vi "Download Dependencies.vi"(5 "Version":string, 7 "Target Directory":path, 8 "error in (no error)":errorcluster, 11 "Platform":T1) -> (0 "error out":errorcluster, 3 "Downloaded File":path)   [LabVIEW 2020, in "binary_installation_tools.lvlib"]
uses:
  binary_installation_tools.lvlib
  Binary Dependency Platform.ctl
  cc709fcc-8e9f-4311-8ae8-324c277baac9.vi
  Get Headers.vi
  <vilib>/security/Message Digest/API/Instances/File/SHA-256 File Checksum.vi
  <vilib>/httpClient/LabVIEWHTTPClient.lvlib
  <vilib>/security/Message Digest/API/NI_Message Digest API.lvlib
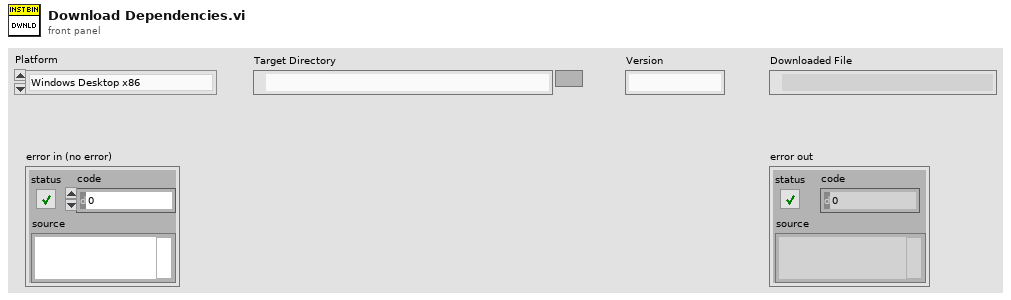
[diagram p1: front panel]
types:
  T1 = typedef "binary_installation_tools.lvlib/Binary Dependency Platform.ctl" = enum16{"Windows Desktop x86", "Windows Desktop x64", "Linux Desktop x64", "Linux Desktop aarch64", "NI Linux RT x64", "NI Linux RT armv7a"}
  T2 = enum16{"Get Manifest", "Check Download in Manifest", "Download", "Verify Checksum"}
  T3 = enum16{"Get Manifest", "Check Download in Manifest", "Download", "Verify Checksum"}[]
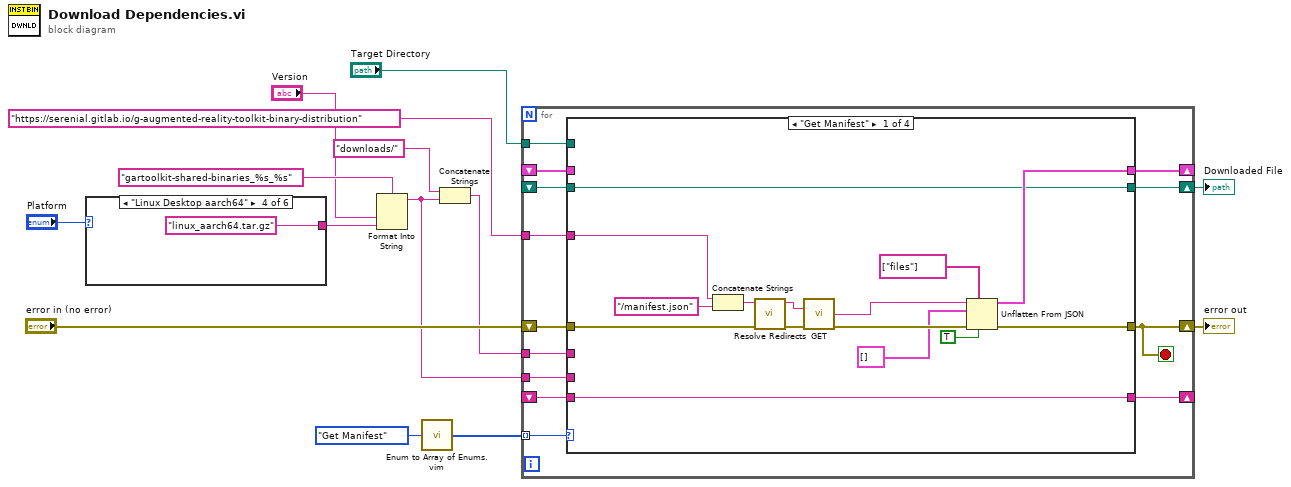
[diagram p0: block diagram]
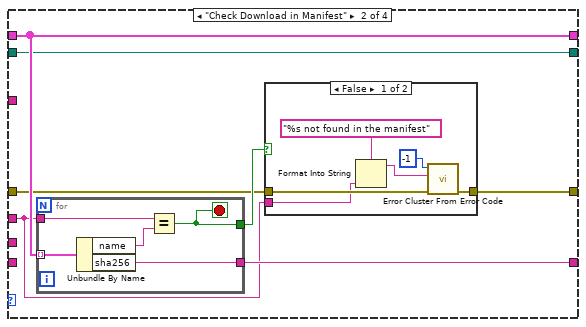
[diagram p2: hidden frame]
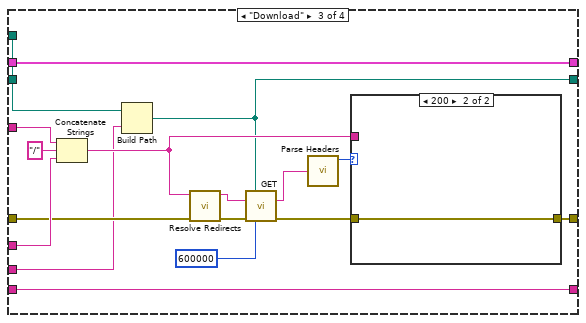
[diagram p4: hidden frame]
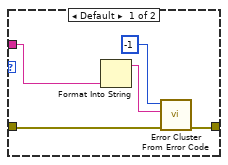
[diagram p5: hidden frame]
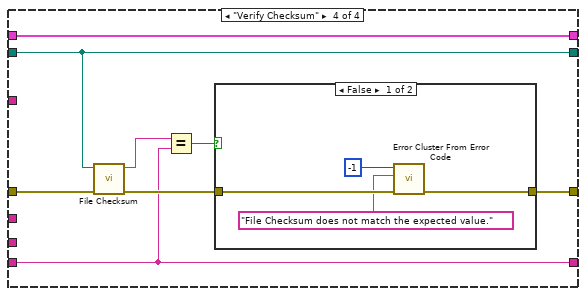
[diagram p6: hidden frame]
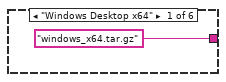
[diagram p8: hidden frame]
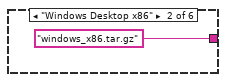
[diagram p9: hidden frame]
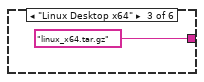
[diagram p10: hidden frame]
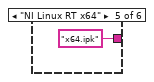
[diagram p11: hidden frame]
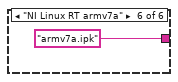
[diagram p12: hidden frame]
diagram:
  n1 = case shown="\"Linux Desktop aarch64\"" "Platform" {
    tunnel: ["windows_x64.tar.gz" "windows_x86.tar.gz" "linux_x64.tar.gz" "linux_aarch64.tar.gz" "x64.ipk" "armv7a.ipk"] -> w8
    frame "Windows Desktop x64" {
    }
    frame "Windows Desktop x86" {
    }
    frame "Linux Desktop x64" {
    }
    frame "Linux Desktop aarch64" {
    }
    frame "NI Linux RT x64" {
    }
    frame "NI Linux RT armv7a" {
    }
  }
  n2 = Format Into String(format string="gartoolkit-shared-binaries_%s_%s", "Version", w8) -> (resulting string=w4:string)  [unwired: 2 in, 1 out]
  n3 = call "Enum to Array of Enums.vim"("enum"=T2."Get Manifest") -> ("array of enums"=w11:T3)
  n4 = Concatenate Strings("downloads/" ("string"), w4) -> (w6:string)
  n5 = for {
    tunnel: w11 -> [w33] mode=indexing
    tunnel: "https://serenial.gitlab.io/g-augmented-reality-toolkit-binary-distribution" -> [w32]
    shift-right: [w25] -> w7
    shift-left: "error in (no error)" -> [w31]
    shift-right: [w30] -> _
    shift-left: _ -> [w29]
    tunnel: w6 -> [w28]
    shift-right: [w27] -> _
    shift-left: _ -> [w26]
    shift-right: [w24] -> w2
    shift-left: _ -> [w23]
    tunnel: w4 -> [w22]
    tunnel: "Target Directory" -> [w21]
    stop <- w25 stop-if-true
    n6 = case shown="\"Get Manifest\"" w33 {
      tunnel: w32 -> [w47 _ w81 _]
      tunnel: w31 -> [w44 w52 w78 w96]
      tunnel: [w38 w51 w72 w91] -> w25
      tunnel: [w36 w55 w84 w98] -> w30
      tunnel: w29 -> [_ w55 w84 w98]
      tunnel: w28 -> [_ w50 w80 _]
      tunnel: [w35 w54 w83 w93] -> w27
      tunnel: w26 -> [w35 _ w83 w93]
      tunnel: [w34 w49 w70 w97] -> w24
      tunnel: w23 -> [w34 w49 _ w97]
      tunnel: w22 -> [_ _ w69 _]
      tunnel: w21 -> [_ _ w68 _]
      frame "Get Manifest" {
        n7 = Concatenate Strings(w47, "/manifest.json" ("string")) -> (w48:string)
        n8 = call "Resolve Redirects.vi"("error in (no error)"=w44, "URL"=w48) -> ("error out"=w43:errorcluster, "URL out"=w45:string)  [unwired: 8 in]
        n9 = call <vilib>:"GET.vi"("url"=w45, "error in (no error)"=w43) -> ("body"=w41:string, "error out"=w42:errorcluster)  [unwired: 10 in, 2 out]
        n10 = Unflatten From JSON(path=string[] ["files"], JSON string=w41, type and defaults=cluster{"name":string, "sha256":string}[] [], default null elements? (F)=TRUE, error in (no error)=w42) -> (value=w36:cluster{"name":string, "sha256":string}[], error out=w38:errorcluster)  [unwired: 2 in]
      }
      frame "Check Download in Manifest" {
        n11 = for {
          tunnel: w50 -> [w60]
          tunnel: w55 -> [w59] mode=indexing
          tunnel: [w57] -> w53
          tunnel: [w56] -> w54
          stop <- w57 stop-if-true
          n12 = Unbundle By Name(w59) -> ("name"=w58:string, "sha256"=w56:string)
          n13 = Equal?(x=w60, y=w58) -> (x = y?=w57:bool)
        }
        n14 = case shown="False" w53 {
          tunnel: w52 -> [w66 w67]
          tunnel: [w65 w67] -> w51
          tunnel: w50 -> [w61 _]
          frame False {
            n15 = Format Into String(format string="%s not found in the manifest" ("error message (\"\")"), w61) -> (resulting string=w62:string)  [unwired: 2 in, 1 out]
            n16 = call <vilib>:"Error Cluster From Error Code.vi"("error in (no error)"=w66, "error message (\"\")"=w62, "error code (0)"=-1) -> ("error out"=w65:errorcluster)  [unwired: 6 in]
          }
          frame True {
          }
        }
      }
      frame "Download" {
        n17 = Concatenate Strings(w81, "/" ("string"), w80) -> (w71:string)
        n18 = Build Path(base path=w68, name or relative path=w69) -> (appended path=w70:path)
        n19 = call "Resolve Redirects.vi"("error in (no error)"=w78, "URL"=w71) -> ("error out"=w77:errorcluster, "URL out"=w82:string)  [unwired: 8 in]
        n20 = call <vilib>:"GET.vi"("output file"=w70, "url"=w82, "error in (no error)"=w77, "timeout (10000)"=600000) -> ("headers"=w75:string, "error out"=w74:errorcluster)  [unwired: 8 in, 2 out]
        n21 = call "Parse Headers.vi"("Headers"=w75) -> ("Response Code"=w73:i32)  [unwired: 3 in, 4 out]
        n22 = case shown="200" w73 {
          tunnel: w74 -> [w88 w90]
          tunnel: [w89 w90] -> w72
          tunnel: w71 -> [w87 _]
          frame Default {
            n23 = Format Into String(w87) -> (resulting string=w86:string)  [unwired: 3 in, 1 out]
            n24 = call <vilib>:"Error Cluster From Error Code.vi"("error in (no error)"=w88, "error message (\"\")"=w86, "error code (0)"=-1) -> ("error out"=w89:errorcluster)  [unwired: 6 in]
          }
          frame 200 {
          }
        }
      }
      frame "Verify Checksum" {
        n25 = call-poly <vilib>:"File Checksum.vi"("error in"=w96, "path"=w97) -> ("error out"=w95:errorcluster, "digest"=w94:string)  [unwired: 8 in]
        n26 = Equal?(x=w94, y=w93) -> (x = y?=w92:bool)
        n27 = case shown="False" w92 {
          tunnel: w95 -> [w101 w103]
          tunnel: [w102 w103] -> w91
          frame False {
            n28 = call <vilib>:"Error Cluster From Error Code.vi"("error in (no error)"=w101, "error message (\"\")"="File Checksum does not match the expected value." ("error message (\"\")"), "error code (0)"=-1) -> ("error out"=w102:errorcluster)  [unwired: 6 in]
          }
          frame True {
          }
        }
      }
    }
  }
  "error out" <- w7
  "Downloaded File" <- w2
